vi "Delete.vi"(8 "error in (no error)":errorcluster, 9 "Parameter":string, 10 "Request":string, 11 "ByteGSWebAPI-V0 in":refnum<class "ByteGSWebAPI-V0.lvclass">) -> (0 "error out":errorcluster, 3 "ByteGSWebAPI-V0 out":refnum<class "ByteGSWebAPI-V0.lvclass">, 4 "body":string, 6 "headers":string)   [LabVIEW 2019, in "ByteGSWebAPI.lvlib" / "ByteGSWebAPI-V0.lvclass"]
uses:
  ByteGSWebAPI-V0.lvclass
  <vilib>/httpClient/LabVIEWHTTPClient.lvlib
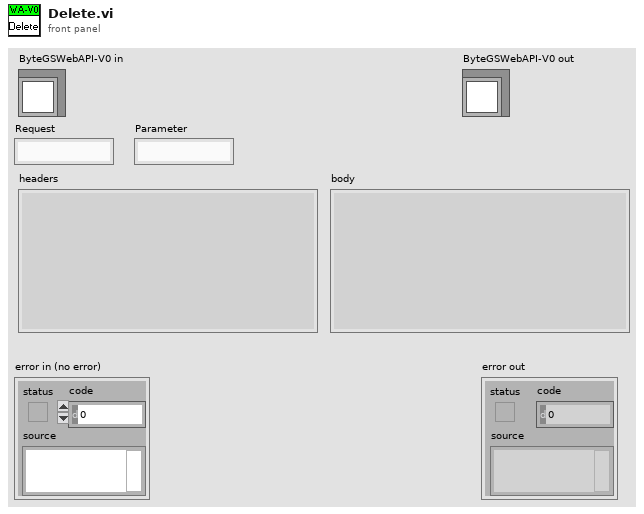
[diagram p1: front panel]
types:
  T1 = typedef "LabVIEWHTTPClient.lvlib/ClientHandle.ctl" = refnum<k1>
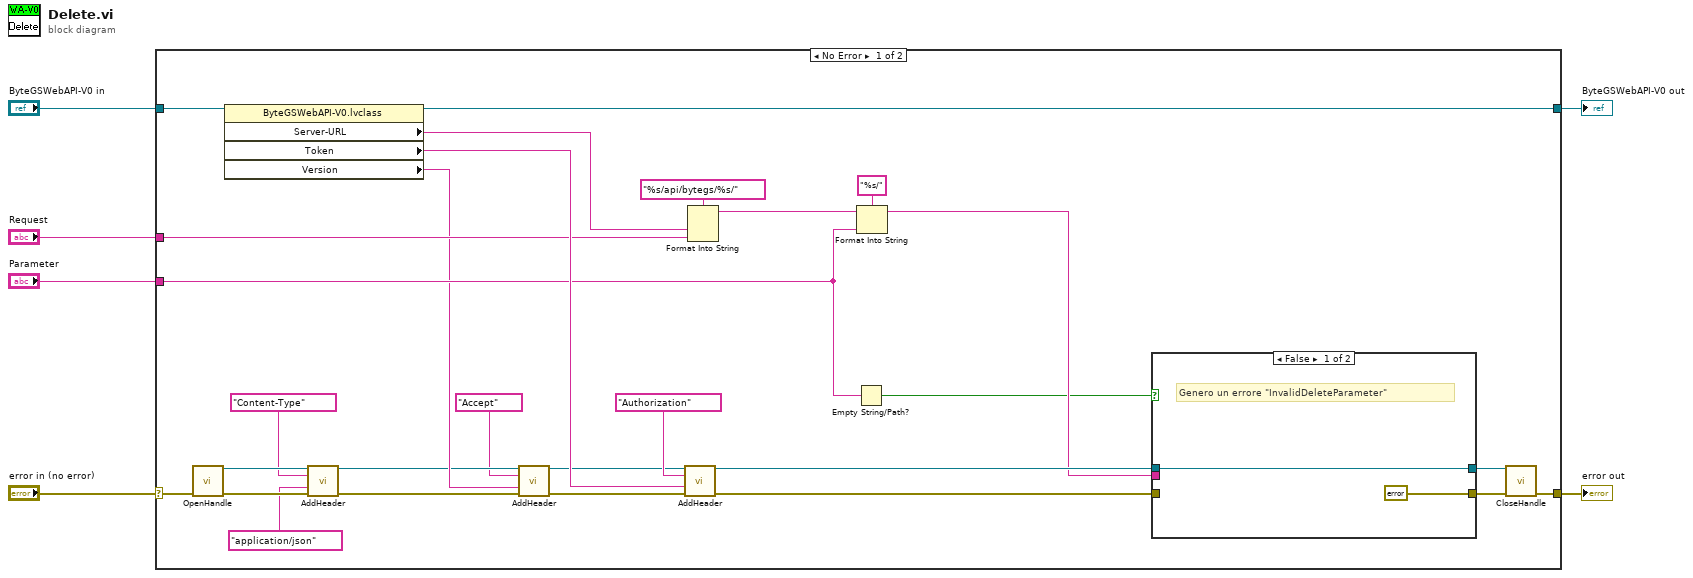
[diagram p0: block diagram]
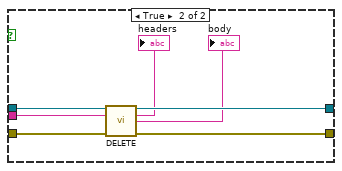
[diagram p2: hidden frame]
diagram:
  n1 = case shown="No Error" "error in (no error)" {
    selector: "error in (no error)" -> [w29 w45]
    tunnel: [w28 w45] -> w5
    tunnel: [w27 w44] -> w3
    tunnel: "ByteGSWebAPI-V0 in" -> [w26 w44]
    tunnel: "Request" -> [w22 _]
    tunnel: "Parameter" -> [w20 _]
    frame No Error {
      n2 = call <vilib>:"OpenHandle.vi"("error in (no error)"=w29) -> ("client handle out"=w32:T1, "error out"=w33:errorcluster)  [unwired: 13 in]
      n3 = property class="ByteGSWebAPI-V0.lvclass"(reference=w26) -> (reference out=w27:refnum<class "ByteGSWebAPI-V0.lvclass">, "Server-URL"=w23:string, "Token"=w25:string, "Version"=w19:string)  [unwired: 1 in, 1 out]
      n4 = call <vilib>:"AddHeader.vi"("client handle"=w32, "header"="Content-Type", "value"="application/json", "error in (no error)"=w33) -> ("client handle out"=w18:T1, "error out"=w17:errorcluster)  [unwired: 10 in]
      n5 = call <vilib>:"AddHeader.vi"("client handle"=w18, "header"="Accept", "value"=w19, "error in (no error)"=w17) -> ("client handle out"=w15:T1, "error out"=w16:errorcluster)  [unwired: 10 in]
      n6 = call <vilib>:"AddHeader.vi"("client handle"=w15, "header"="Authorization", "value"=w25, "error in (no error)"=w16) -> ("client handle out"=w13:T1, "error out"=w11:errorcluster)  [unwired: 10 in]
      n7 = Format Into String(format string="%s/api/bytegs/%s/" ("url"), w23, w22) -> (resulting string=w21:string)  [unwired: 2 in, 1 out]
      n8 = Empty String/Path?(string/path=w20) -> (empty?=w7:bool)
      n9 = Format Into String(format string="%s/" ("url"), initial string=w21, w20) -> (resulting string=w9:string)  [unwired: 1 in, 1 out]
      n10 = case shown="False" w7 {
        tunnel: w13 -> [w36 w43]
        tunnel: [w36 w42] -> w12
        tunnel: w11 -> [_ w41]
        tunnel: [errorcluster {"status"=TRUE, "code"=10, "source"="InvalidDeleteParameter"} ("error out") w40] -> w10
        tunnel: w9 -> [_ w37]
        frame False {
          # "Genero un errore \"InvalidDeleteParameter\""
        }
        frame True {
          n11 = call <vilib>:"DELETE.vi"("client handle"=w43, "url"=w37, "error in (no error)"=w41) -> ("client handle out"=w42:T1, "headers"=→"headers":string, "body"=→"body":string, "error out"=w40:errorcluster)  [unwired: 9 in]
        }
      }
      n12 = call <vilib>:"CloseHandle.vi"("client handle"=w12, "error in (no error)"=w10) -> ("error out"=w28:errorcluster)  [unwired: 13 in]
    }
    frame Error {
    }
  }
  "error out" <- w5
  "ByteGSWebAPI-V0 out" <- w3
